vi "PJT_04.vi"() -> ()   [LabVIEW 2019]
panel:
  out "길이":i32
  out "연결된 문자열":string
  in  "문자열":string
  in  "입력 1":dbl
  in  "초기 문자열":string
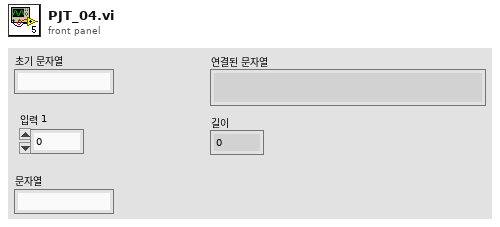
[diagram p1: front panel]
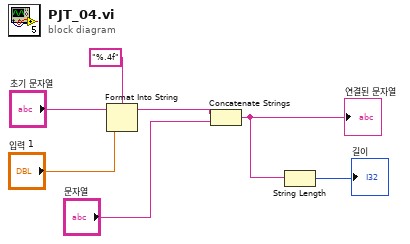
[diagram p0: block diagram]
diagram:
  n1 = Format Into String(format string="%.4f" ("포맷 문자열"), initial string="초기 문자열", "입력 1") -> (resulting string=w5:string)  [unwired: 1 in, 1 out]
  n2 = Concatenate Strings(w5, "문자열") -> (w2:string)
  "연결된 문자열" <- w2
  n3 = String Length(string=w2) -> (length=→"길이":i32)
